vi "AjouterLivraison.vi"(1 "date livraison":string, 2 "num_cmd":string, 3 "?":bool) -> ()   [LabVIEW 2024]
uses:
  <vilib>/drjdpowell/SQLite Library/SQL Connection/Open (string).vi
  <vilib>/drjdpowell/SQLite Library/SQL Connection/Execute SQL.vi
  <vilib>/drjdpowell/SQLite Library/SQL Connection/Connection.lvclass
  <vilib>/drjdpowell/SQLite Library/SQLite.lvlib
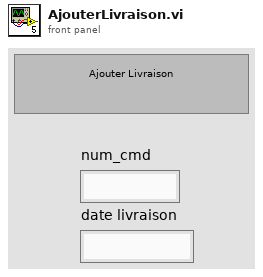
[diagram p1: front panel]
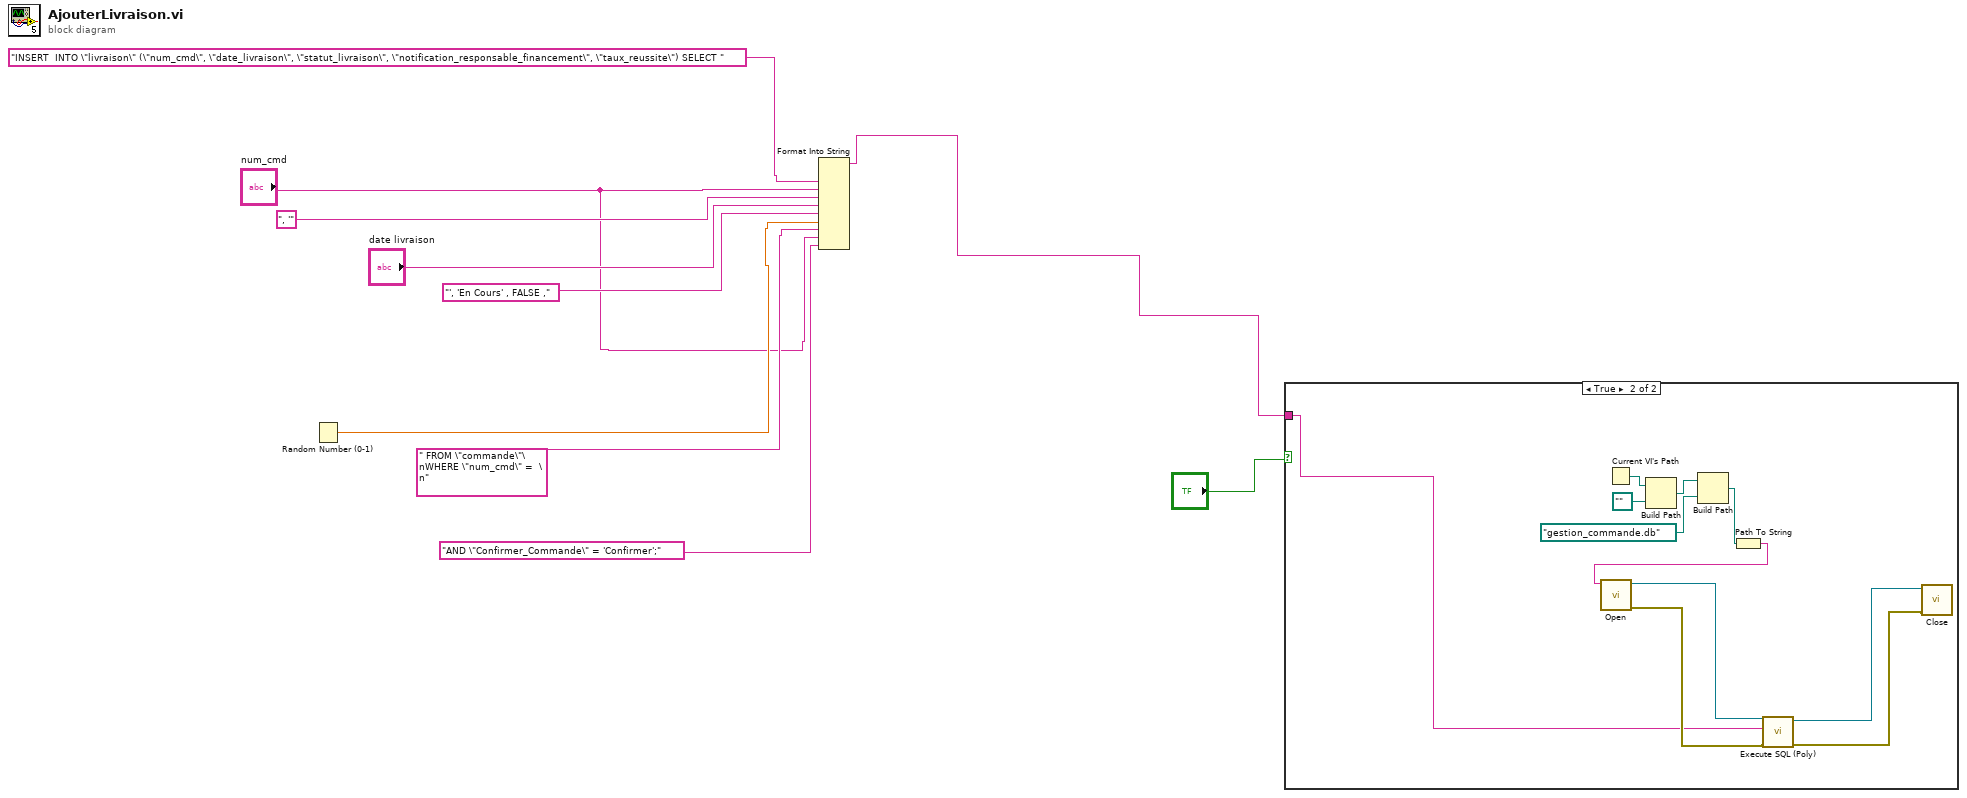
[diagram p0: block diagram]
diagram:
  n1 = Random Number (0-1)() -> (number: 0 to 1=w7:dbl)
  n2 = Format Into String("INSERT  INTO \"livraison\" (\"num_cmd\", \"date_livraison\", \"statut_livraison\", \"notification_responsable_financement\", \"taux_reussite\") SELECT " ("SQL"), "num_cmd", ", '", "date livraison", "', 'En Cours' , FALSE ,", w7, " FROM \"commande\"\nWHERE \"num_cmd\" =  \n", "num_cmd", "AND \"Confirmer_Commande\" = 'Confirmer';") -> (resulting string=w1:string)  [unwired: 3 in, 1 out]
  n3 = case shown="True" "?" {
    tunnel: w1 -> [_ w17]
    frame False {
    }
    frame True {
      n4 = Current VI's Path() -> (path=w16:path)
      n5 = Build Path(base path=w16, name or relative path=path "..") -> (appended path=w13:path)
      n6 = Build Path(base path=w13, name or relative path=path "gestion_commande.db" ("Filename")) -> (appended path=w12:path)
      n7 = Path To String(path=w12) -> (string=w11:string)
      n8 = call-poly <vilib>:"Open.vi"("db file"=w11) -> ("error out"=w21:errorcluster, "SQLite Connection"=w18:refnum<class "Connection.lvclass">)  [unwired: 9 in]
      n9 = call-poly <vilib>:"Execute SQL (Poly).vi"("error in (no error)"=w21, "SQL"=w17, "SQLite Connection in"=w18) -> ("error out"=w20:errorcluster, "SQLite Connection"=w19:refnum<class "Connection.lvclass">)  [unwired: 5 in, 2 out]
      n10 = call-dynamic "Close.vi"("error in (no error)"=w20, "SQLite Connection in"=w19) -> ()  [unwired: 9 in, 1 out]
    }
  }
